vi "GetSingleMeasurementDemo.vi"() -> ()   [LabVIEW 2016]
doc: "This VI demonstrates how to get measurement values without starting a continuous measurement. \nMeasuremet values are obtained by a repeated calling of the GetSingleMeasurementValue vi."
panel:
  out "Diagram":waveform(dbl)[](graph)
  in  "?":bool
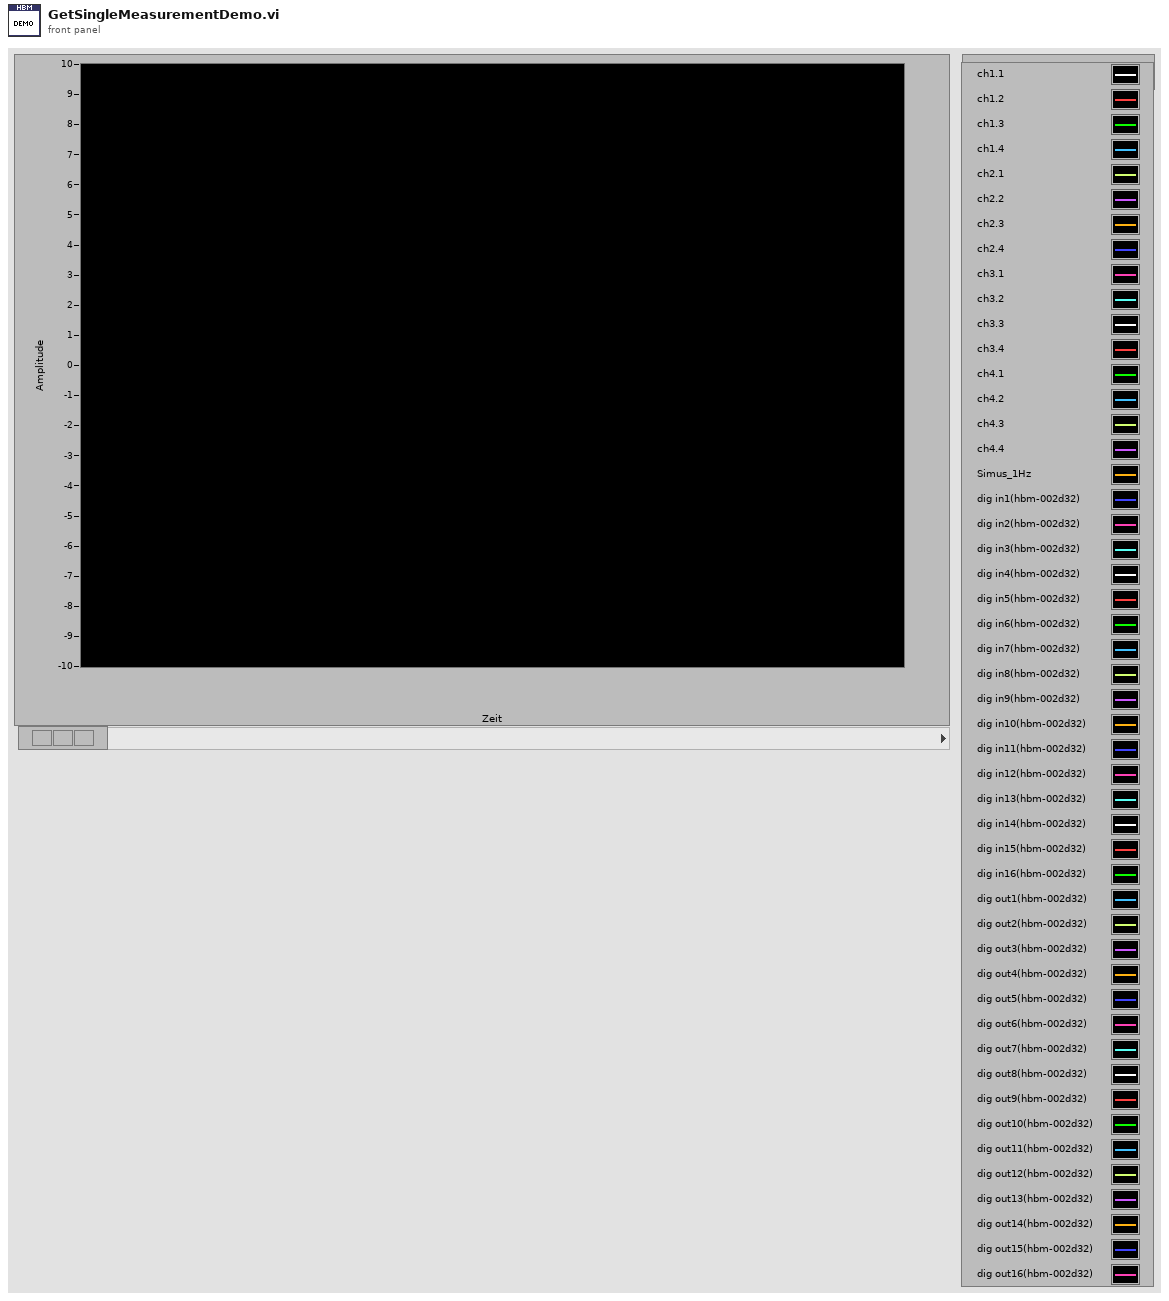
[diagram p1: front panel]
types:
  T1 = cluster{"Devices":refnum<k24>[], "Signals":refnum<k24>[]}
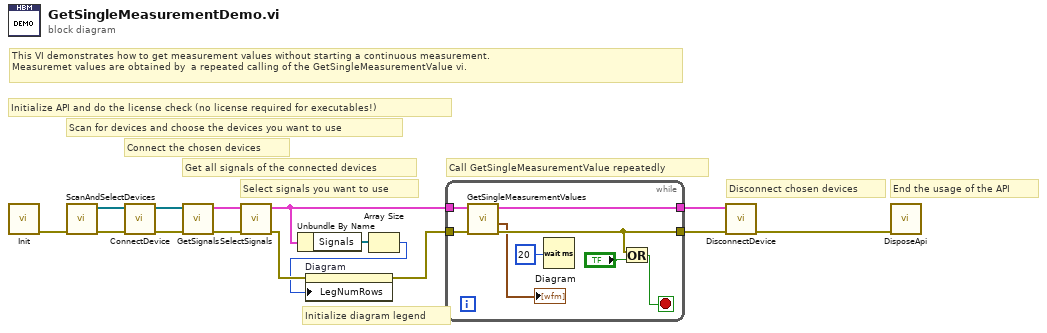
[diagram p0: block diagram]
diagram:
  # "Disconnect chosen devices"
  # "Call GetSingleMeasurementValue repeatedly"
  # "Initialize diagram legend"
  # "End the usage of the API"
  # "This VI demonstrates how to get measurement values without starting a continuous measurement. \nMeasuremet values are obtained by  a repeated calling of the GetSingleMeasurementValue vi."
  # "Select signals you want to use"
  # "Get all signals of the connected devices"
  # "Connect the chosen devices"
  # "Scan for devices and choose the devices you want to use"
  # "Initialize API and do the license check (no license required for executables!)"
  n1 = call "Init.vi"() -> ("Error out"=w9:errorcluster)  [unwired: 8 in, 2 out]
  n2 = call "ScanAndSelectDevices.vi"("Error in"=w9) -> ("Error out"=w15:errorcluster, "SelectedDevices"=w12:refnum<k24>[])  [unwired: 8 in, 1 out]
  n3 = call "ConnectDevice.vi"("Error in"=w15, "Devices"=w12) -> ("Error out"=w14:errorcluster, "Devices"=w11:refnum<k24>[])  [unwired: 7 in, 1 out]
  n4 = call "GetSignals.vi"("Error in"=w14, "Devices"=w11) -> ("Error out"=w13:errorcluster, "DevicesAndSignals"=w10:T1)  [unwired: 7 in, 1 out]
  n5 = call "SelectSignals.vi"("error in (no error)"=w13, "DevicesAndSignals"=w10) -> ("error out"=w6:errorcluster, "DevicesAndSignals"=w8:T1)  [unwired: 7 in, 1 out]
  n6 = Unbundle By Name(w8) -> ("Signals"=w7:refnum<k24>[])
  n7 = Array Size(array=w7) -> (size(s)=w5:i32)
  n8 = property on="Diagram" class="WFChart (严格)"(error in=w6, "LegNumRows"=w5) -> (error out=w4:errorcluster)  [unwired: 1 in, 1 out]
  n9 = while {
    tunnel: w8 -> [w23]
    tunnel: w4 -> [w22]
    tunnel: [w21] -> w3
    tunnel: [w17] -> w1
    stop <- w19 stop-if-true
    n10 = call "GetSingleMeasurementValues.vi"("Error in"=w22, "DevicesAndSignals"=w23) -> ("Error out"=w21:errorcluster, "MeasurementValues(Waveform)"=→"Diagram":waveform(dbl)[], "DevicesAndSignals"=w17:T1)  [unwired: 7 in]
    n11 = Wait (ms)(milliseconds to wait=u32 20 ("Zu wartende ms")) -> ()  [unwired: 1 out]
    n12 = Or(x=w21, y="?") -> (x .or. y?=w19:bool)
  }
  n13 = call "DisconnectDevice.vi"("Error in"=w3, "DevicesAndSignals"=w1) -> ("Error out"=w2:errorcluster)  [unwired: 9 in]
  n14 = call "DisposeApi.vi"("Error in"=w2) -> ()  [unwired: 10 in, 1 out]
